vi "SetResultCluster.vi"(9 "data":string[](array[string]), 10 "测试结果簇":refnum<vi>) -> ()   [LabVIEW 2013]
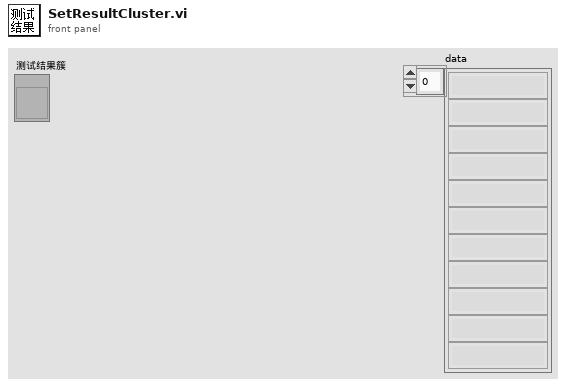
[diagram p1: front panel]
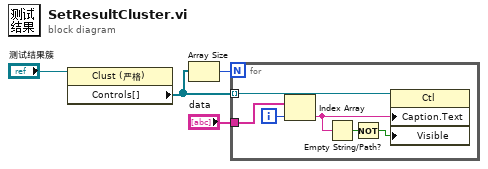
[diagram p0: block diagram]
diagram:
  n1 = property class="Clust (严格)"(reference="测试结果簇") -> ("Controls[]"=w3:refnum<vi>[])  [unwired: 1 in, 2 out]
  n2 = Array Size(array=w3) -> (size(s)=w2:i32)
  n3 = for {
    N: w2 -> [_]
    tunnel: w3 -> [w10] mode=indexing
    tunnel: "data" -> [w9]
    i -> [w8]
    n4 = Index Array(array=w9, index=w8) -> (element=w7:string)
    n5 = Empty String/Path?(string/path=w7) -> (empty?=w6:bool)
    n6 = Not(x=w6) -> (.not. x?=w5:bool)
    n7 = property class="Ctl"(reference=w10, "Caption.Text"=w7, "Visible"=w5) -> ()  [unwired: 1 in, 2 out]
  }
